vi "VISA_Exemple.vi"() -> ()   [LabVIEW 2019]
uses:
  <vilib>/Instr/_visa.llb/VISA Configure Serial Port (Instr).vi
panel:
  in  "Enable Termination\nChar (T)":bool=TRUE
  in  "Stop Button":bool
  out "Numeric Indicator":dbl format="%#_9g"
  out "Waveform Chart":i32(graph)
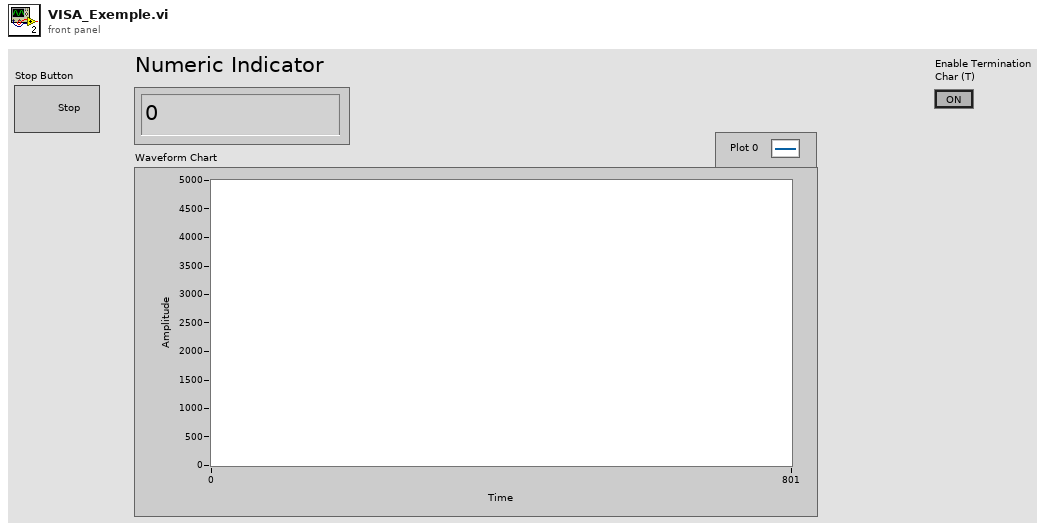
[diagram p1: front panel]
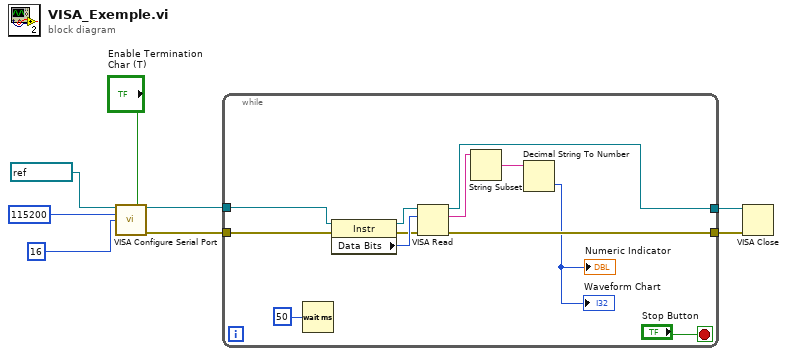
[diagram p0: block diagram]
diagram:
  n1 = call-poly "VISA Configure Serial Port"("VISA resource name"=refnum<visa-resource-name> "COM3" ("COM Port"), "Enable Termination\nChar (T)"="Enable Termination\nChar (T)", "baud rate (9600)"=u32 115200, "data bits (8)"=u16 16) -> ("VISA resource name out"=w5:refnum<visa-resource-name>, "error out"=w4:errorcluster)  [unwired: 10 in]
  n2 = while {
    tunnel: [w20] -> w7
    tunnel: [w19] -> w6
    tunnel: w5 -> [w18]
    tunnel: w4 -> [w17]
    stop <- "Stop Button" stop-if-true
    n3 = Wait (ms)(milliseconds to wait=u32 50) -> ()  [unwired: 1 out]
    n4 = property class="Instr"(reference=w18, error in=w17) -> (reference out=w14:refnum<visa-resource-name>, error out=w15:errorcluster, "Data Bits"=w16:u16)
    n5 = VISA Read(VISA resource name=w14, byte count=w16, error in (no error)=w15) -> (VISA resource name out=w20:refnum<visa-resource-name>, read buffer=w11:string, error out=w19:errorcluster)  [unwired: 1 out]
    n6 = String Subset(string=w11) -> (substring=w13:string)  [unwired: 2 in]
    n7 = Decimal String To Number(string=w13) -> (number=→"Waveform Chart" →"Numeric Indicator":i32)  [unwired: 2 in, 1 out]
  }
  n8 = VISA Close(VISA resource name=w7, error in (no error)=w6) -> ()  [unwired: 1 out]
